vi "ppanel_process_error.vi"(8 "error in (no error)":errorcluster, 9 "update_status":bool=TRUE, 10 "No Error Message":string, 11 "hydraharp_panel in":refnum<class "picoharp_panel.lvclass">) -> (0 "error out":errorcluster, 3 "hydraharp_panel out":refnum<class "picoharp_panel.lvclass">)   [LabVIEW 2015, in "picoharp_panel.lvclass"]
uses:
  picoharp_panel.lvclass
  Hydraharp/hydraharp_panel/hpanel_messages_to_panel_from_actor_loop.ctl
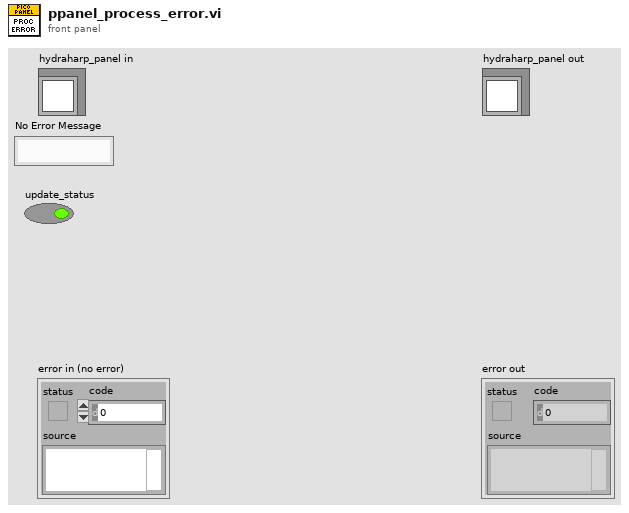
[diagram p1: front panel]
types:
  T1 = typedef "hpanel_messages_to_panel_from_actor_loop.ctl" = enum16{"reenable_tasks"}
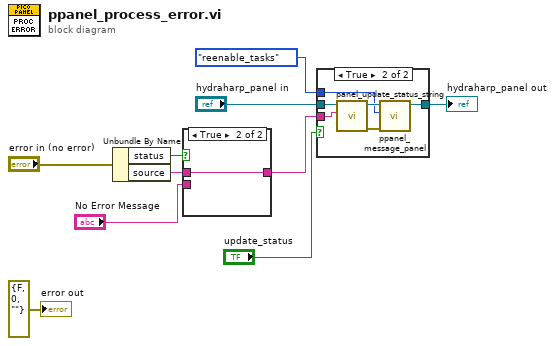
[diagram p0: block diagram]
diagram:
  n1 = Unbundle By Name("error in (no error)") -> ("status"=w7:bool, "source"=w4:string)
  n2 = case shown="True" w7 {
    tunnel: "No Error Message" -> [w11 _]
    tunnel: [w11 w12] -> w5
    tunnel: w4 -> [_ w12]
    frame False {
    }
    frame True {
    }
  }
  n3 = case shown="True" "update_status" {
    tunnel: "hydraharp_panel in" -> [w13 w19]
    tunnel: hpanel_messages_to_panel_from_actor_loop."reenable_tasks" ("event data") -> [_ w15]
    tunnel: w5 -> [_ w14]
    tunnel: [w13 w18] -> w1
    frame False {
    }
    frame True {
      n4 = call-dynamic "panel_update_status_string.vi"("String"=w14, "hydraharp_panel in"=w19) -> ("error out"=w17:errorcluster, "hydraharp_panel out"=w16:refnum<class "picoharp_panel.lvclass">)  [unwired: 8 in]
      n5 = call "ppanel_message_panel.vi"("error in (no error)"=w17, "event data"=w15, "hydraharp_panel in"=w16) -> ("hydraharp_panel out"=w18:refnum<class "picoharp_panel.lvclass">)  [unwired: 7 in, 1 out]
    }
  }
  "hydraharp_panel out" <- w1
  "error out" <- errorcluster {"status"=FALSE, "code"=0, "source"=""} ("error out")
